vi "test-path-planner-basic.vi"() -> ()   [LabVIEW 2019]
uses:
  <vilib>/Rock Robotics/WPI/ThirdParty/MJansen/PathPlanner/TypeDef/PathPlannerTrajectoryState.ctl
  <vilib>/Rock Robotics/WPI/ThirdParty/JAS_Junk/TrajLib/TypeDef/TRANSLATION2D.ctl
  <vilib>/Rock Robotics/WPI/ThirdParty/JAS_Junk/TrajLib/TypeDef/ROTATION2D.ctl
  <vilib>/Rock Robotics/WPI/ThirdParty/MJansen/PathPlanner/TypeDef/PathPlannerPathConstraints.ctl
  <vilib>/Rock Robotics/WPI/ThirdParty/JAS_Junk/TrajLib/TypeDef/TRAJ_STATE.ctl
  <vilib>/Rock Robotics/WPI/ThirdParty/JAS_Junk/TrajLib/TypeDef/POSE2D.ctl
  <vilib>/Rock Robotics/WPI/ThirdParty/MJansen/PathPlanner/TypeDef/PathPlannerTrajectory.ctl
  <vilib>/Rock Robotics/WPI/ThirdParty/JAS_Junk/TrajLib/Util_ApproxEquals.vi
  <vilib>/Rock Robotics/WPI/ThirdParty/JAS_Junk/TrajLib/TrajectoryState_Equals.vi
  <vilib>/Rock Robotics/WPI/ThirdParty/JAS_Junk/TrajLib/Pose2d_Equals.vi
  <vilib>/Rock Robotics/WPI/ThirdParty/JAS_Junk/TrajLib/Translation2d_Equals.vi
  <vilib>/Rock Robotics/WPI/ThirdParty/JAS_Junk/TrajLib/Rotation2d_Equals.vi
  <vilib>/Rock Robotics/WPI/ThirdParty/JAS_Junk/TrajLib/Util_CalcDist.vi
  <vilib>/Rock Robotics/WPI/ThirdParty/MJansen/PathPlanner/PathPlanner24.lvlib
  <vilib>/Rock Robotics/WPI/ThirdParty/JAS_Junk/TrajLib/Trajectory_Library.lvlib
  <vilib>/Analysis/NI_AALBase.lvlib
panel:
  out "PathPlannerTrajectory":T1 {"States"."TargetHolonomicRotation"."SIN" format="%13.4f"; "States"."TargetHolonomicRotation"."COS" format="%13.4f"; "States"."TargetHolonomicRotation"."VALUE" format="%13.4f"; "States"."Heading"."SIN" format="%13.4f"; "States"."Heading"."COS" format="%13.4f"; "States"."Heading"."VALUE" format="%13.4f"; "States"."PositionMeters"."Y" format="%14.3f"; "States"."PositionMeters"."X" format="%14.3f"}
  in  "Tab Control":T6(tab)
  in  "jsonReadTrajFile":string="C:\\Shares\\github\\PathPlannerLabVIEW\\PathPlannerSandbox\\PathPlannerTestPath\\Javapath1.json"
  in  "stop":bool
  in  "Path FileName":string="C:\\Shares\\github\\PathPlannerLabVIEW\\PathPlannerSandbox\\PathPlannerTestPath\\jim1.PATH"
  out "LabVIEW path json read error":errorcluster
  in  "LabVIEW jsonWriteFile":string="C:\\Shares\\github\\PathPlannerLabVIEW\\PathPlannerSandbox\\PathPlannerTestPath\\LabVIEWpath1.json"
  out "Java File Read Error":errorcluster
  out "LabView Write\nJSON Error":errorcluster
  out "outPathPlannerStates":T2[](array[typedef]) {"TargetHolonomicRotation"."SIN" format="%13.4f"; "TargetHolonomicRotation"."COS" format="%13.4f"; "TargetHolonomicRotation"."VALUE" format="%13.4f"; "Heading"."SIN" format="%13.4f"; "Heading"."COS" format="%13.4f"; "Heading"."VALUE" format="%13.4f"; "PositionMeters"."Y" format="%14.3f"; "PositionMeters"."X" format="%14.3f"}
  in  "Down Button":bool
  in  "Up Button":bool
  in  "index":i32 step=20
  out "Java_TotalTime_Sec":dbl
  out "LabVIEW_TotalTime_Sec":dbl
  out "Jave and LabVIEW \nexactly equal":bool
  out "JavaStateCount":i32
  out "LabVIEWStateCount":i32
  out "States Check":bool[](array[boolean])
  out "JavaStates":T7[](array[typedef]) {"POSE"."ROTATION"."SIN" format="%13.4f"; "POSE"."ROTATION"."COS" format="%13.4f"; "POSE"."ROTATION"."VALUE" format="%13.4f"; "POSE"."TRANSLATION"."Y" format="%14.3f"; "POSE"."TRANSLATION"."X" format="%14.3f"}
  out "LabVIEWStates":T7[](array[typedef]) {"POSE"."ROTATION"."SIN" format="%13.4f"; "POSE"."ROTATION"."COS" format="%13.4f"; "POSE"."ROTATION"."VALUE" format="%13.4f"; "POSE"."TRANSLATION"."Y" format="%14.3f"; "POSE"."TRANSLATION"."X" format="%14.3f"}
  out "Differences":T7[](array[typedef]) {"POSE"."ROTATION"."SIN" format="%13.4f"; "POSE"."ROTATION"."COS" format="%13.4f"; "POSE"."ROTATION"."VALUE" format="%13.4f"; "POSE"."TRANSLATION"."Y" format="%14.3f"; "POSE"."TRANSLATION"."X" format="%14.3f"}
  out "max time diff":dbl
  out "max vel diff":dbl
  out "max accel diff":dbl
  out "max x diff":dbl
  out "max y diff":dbl
  out "max rot diff rad":dbl
  out "max curvature diff":dbl
  out "vel mean":dbl format="%0.6f"
  out "vel std dev":dbl format="%0.6f"
  out "accel mean":dbl format="%0.6f"
  out "accel std dev":dbl format="%0.6f"
  out "Java and LabVIEW \nwithin tolerance":bool
  in  "Tolerance":T7={"TimeSeconds"=0.15, "Velocity"=0.25, "Acceleration"=2.5, "POSE"={"TRANSLATION"={"X"=0.015, "Y"=0.015}, "ROTATION"={"VALUE"=0.01, "COS"=0.0, "SIN"=0.0}}, "Curvature"=1.4} {"POSE"."ROTATION"."SIN" format="%13.4f"; "POSE"."ROTATION"."COS" format="%13.4f"; "POSE"."ROTATION"."VALUE" format="%13.4f"; "POSE"."TRANSLATION"."Y" format="%14.3f"; "POSE"."TRANSLATION"."X" format="%14.3f"}
  out "XY SPLINE":cluster{dbl[], dbl[]}[](graph)
  out "XY Graph":cluster{dbl[], dbl[]}[](graph)
  out "Sample Graph":dbl[][](graph)
  out "LabVIEW Time Plot":cluster{dbl[], dbl[]}[](graph)
  out "Java Time Plot":cluster{dbl[], dbl[]}[](graph)
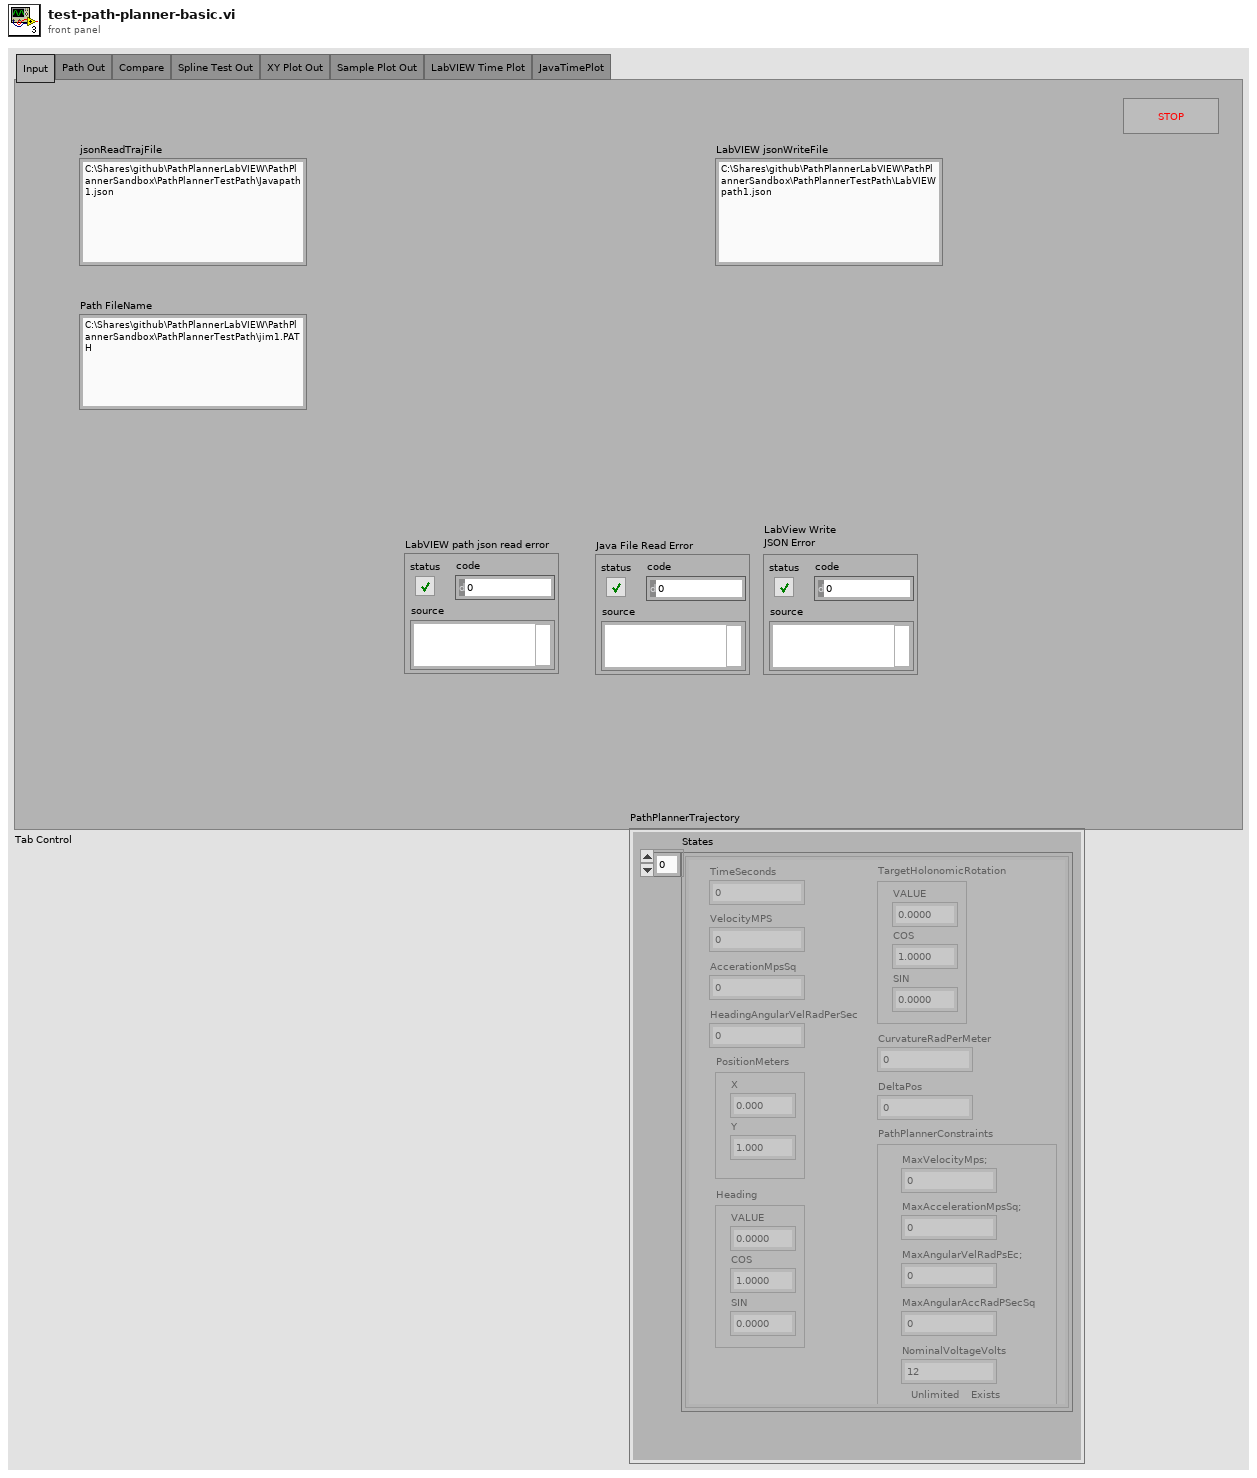
[diagram p1: front panel]
types:
  T1 = typedef "PathPlanner24.lvlib/PathPlannerTrajectory.ctl" = cluster{"States":T2[]}
  T2 = typedef "PathPlanner24.lvlib/PathPlannerTrajectoryState.ctl" = cluster{"TimeSeconds":dbl, "VelocityMPS":dbl, "AccerationMpsSq":dbl, "HeadingAngularVelRadPerSec":dbl, "PositionMeters":T3, "Heading":T4, "TargetHolonomicRotation":T4, "CurvatureRadPerMeter":dbl, "PathPlannerConstraints":T5, "DeltaPos":dbl}
  T3 = typedef "Trajectory_Library.lvlib/TRANSLATION2D.ctl" = cluster{"X":dbl, "Y":dbl}
  T4 = typedef "Trajectory_Library.lvlib/ROTATION2D.ctl" = cluster{"VALUE":dbl, "COS":dbl, "SIN":dbl}
  T5 = typedef "PathPlanner24.lvlib/PathPlannerPathConstraints.ctl" = cluster{"MaxVelocityMps;":dbl, "MaxAccelerationMpsSq;":dbl, "MaxAngularVelRadPsEc;":dbl, "MaxAngularAccRadPSecSq":dbl, "Exists":bool, "Unlimited":bool, "NominalVoltageVolts":dbl}
  T6 = enum32{"Input", "Path Out", "Compare", "Spline Test Out", "XY Plot Out", "Sample Plot Out", "LabVIEW Time Plot", "JavaTimePlot"}
  T7 = typedef "Trajectory_Library.lvlib/TRAJ_STATE.ctl" = cluster{"TimeSeconds":dbl, "Velocity":dbl, "Acceleration":dbl, "POSE":T8, "Curvature":dbl}
  T8 = typedef "Trajectory_Library.lvlib/POSE2D.ctl" = cluster{"TRANSLATION":T3, "ROTATION":T4}
  T9 = typedef "PathPlanner24.lvlib/PathPlannerPath.ctl" = cluster{"Reversed":bool, "RotationTargets":T10[], "ConstraintZones":T11[], "EventMarkers":T12[], "GlobalConstraints":T5, "GoalEndState":T15, "AllPoints":T16[], "Name":string, "Waypoints":T17[], "PointTowardsZones":T18[], "IdealStartingState":T19, "IsChoreoPath":bool, "PreventFlipping":bool}
  T10 = typedef "PathPlanner24.lvlib/PathPlannerRotationTarget.ctl" = cluster{"position":dbl, "rotation":T4, "Exists":bool}
  T11 = typedef "PathPlanner24.lvlib/PathPlannerConstraintsZone.ctl" = cluster{"minPosition":dbl, "maxPosition":dbl, "Constraints":T5, "Present":bool}
  T12 = typedef "PathPlanner24.lvlib/PathPlannerEventMarker.ctl" = cluster{"Position":dbl, "Command":T13, "TriggerName":string, "EndPosition":dbl}
  T13 = typedef "PathPlanner24.lvlib/PathPlannerCommandUtil.ctl" = cluster{"waitTime":dbl, "name":string, "pathName":string, "commands":cluster{"type":T14, "waitTime":dbl, "name":string, "pathName":string}[], "type":T14}
  T14 = typedef "PathPlanner24.lvlib/PathPlanner_CommandUtilType_ENUM.ctl" = enum16{"Unknown", "Wait", "Named", "Path", "Sequential", "Parallel", "Race", "Deadline"}
  T15 = typedef "PathPlanner24.lvlib/PathPlannerGoalEndState.ctl" = cluster{"VelocityMPS":dbl, "Rotation":T4}
  T16 = typedef "PathPlanner24.lvlib/PathPlannerPathPoint.ctl" = cluster{"Position":T3, "DistAlongPath":dbl, "MaxV":dbl, "Constraints":T5, "RotationTarget":T10, "WaypointRelativePos":dbl}
  T17 = typedef "PathPlanner24.lvlib/PathPlannerWaypoint.ctl" = cluster{"prevControl":T3, "anchor":T3, "nextControl":T3, "PrevExists":bool, "NextExists":bool}
  T18 = typedef "PathPlanner24.lvlib/PathPlannerPointTowardsZone.ctl" = cluster{"RotationOffset":T4, "Name":string, "TargetPosition":T3, "MinPosition":dbl, "MaxPosition":dbl}
  T19 = typedef "PathPlanner24.lvlib/PathPlannerIdealStartingState.ctl" = cluster{"VelocityMPS":dbl, "Rotation":T4}
  T20 = typedef "Trajectory_Library.lvlib/TRAJECTORY.ctl" = cluster{"TotalTImeSecs":dbl, "States":T7[]}
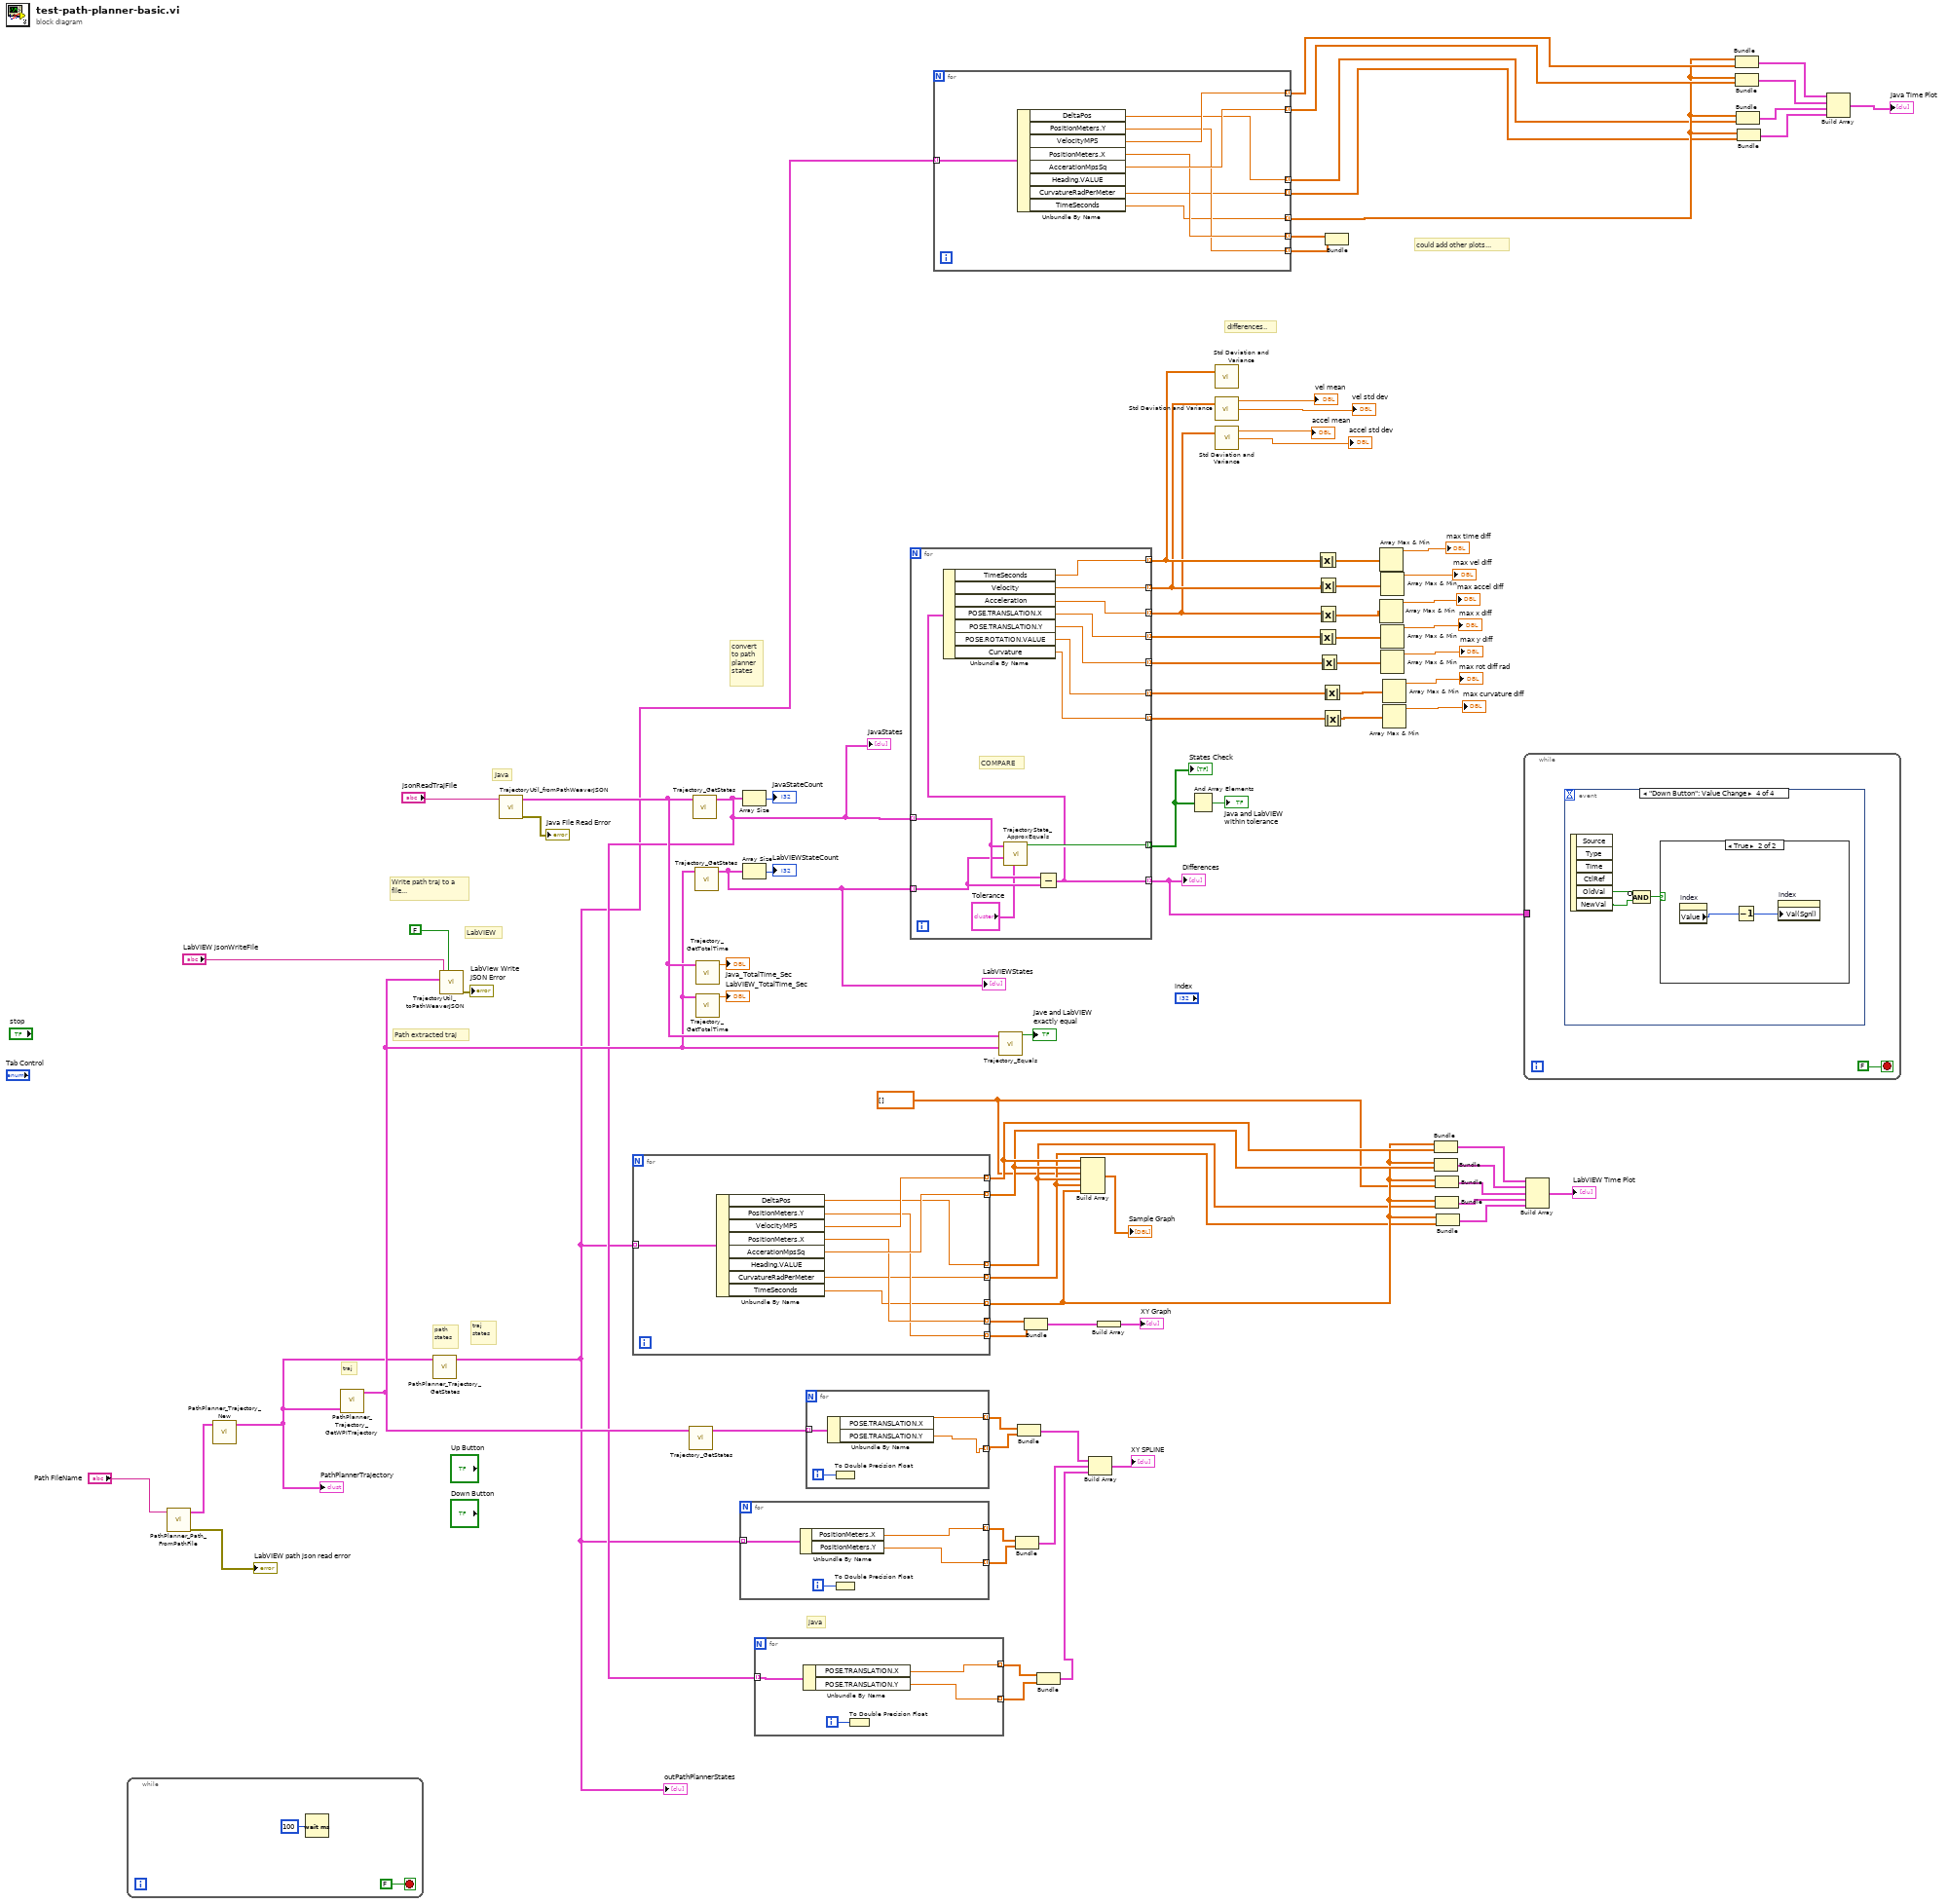
[diagram p0: block diagram]
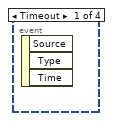
[diagram p2: hidden frame]
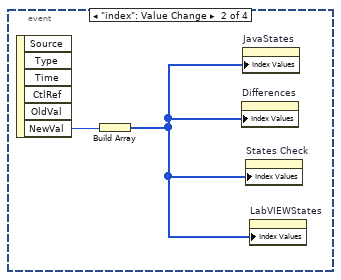
[diagram p3: hidden frame]
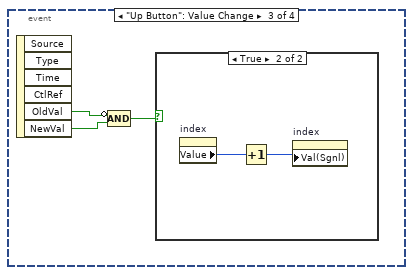
[diagram p4: hidden frame]
diagram:
  w2 = dbl[] [] ("element")
  # "Write path traj to a \nfile..."
  # "Path extracted traj"
  # "traj"
  # "traj\nstates"
  # "path\nstates"
  # "differences.."
  # "could add other plots..."
  # "convert\nto path\nplanner\nstates"
  # "java"
  # "LabVIEW"
  # "Java"
  n1 = while {
    stop <- FALSE stop-if-true
    n2 = Wait (ms)(milliseconds to wait=u32 100) -> ()  [unwired: 1 out]
  }
  n3 = call <vilib>:"PathPlanner_Path_FromPathFile.vi"("FileName"="Path FileName") -> ("error out"=→"LabVIEW path json read error":errorcluster, "PathPlannerPath"=w4:T9)  [unwired: 7 in, 2 out]
  n4 = call <vilib>:"PathPlanner_Trajectory_New.vi"("Path"=w4) -> ("PathPlannerTrajectory"=w3:T1)  [unwired: 9 in, 1 out]
  "PathPlannerTrajectory" <- w3
  n5 = call <vilib>:"PathPlanner_Trajectory_GetWPITrajectory.vi"("PathPlannerTrajectory"=w3) -> ("WPI TRAJECTORY"=w62:T20)  [unwired: 9 in, 1 out]
  n6 = call <vilib>:"PathPlanner_Trajectory_GetStates.vi"("PathPlannerTrajectory"=w3) -> ("PathPlannerStates"=w1:T2[])  [unwired: 10 in]
  "outPathPlannerStates" <- w1
  n7 = call <vilib>:"TrajectoryUtil_toPathWeaverJSON.vi"("AlwaysOverWrite"=FALSE, "inTRAJECTORY"=w62, "FileName"="LabVIEW jsonWriteFile") -> ("error out"=→"LabView Write\nJSON Error":errorcluster)  [unwired: 7 in, 1 out]
  n8 = call <vilib>:"TrajectoryUtil_fromPathWeaverJSON.vi"("FileName"="jsonReadTrajFile") -> ("error out"=→"Java File Read Error":errorcluster, "outTRAJECTORY"=w63:T20)  [unwired: 8 in, 1 out]
  n9 = for {
    tunnel: [w97] -> w31 mode=indexing
    tunnel: [w96] -> w30 mode=indexing
    tunnel: [w91] -> w28 mode=indexing
    tunnel: [w95] -> w86 mode=indexing
    tunnel: [w94] -> w85 mode=indexing
    tunnel: w1 -> [w93] mode=indexing
    tunnel: [w92] -> w27 mode=indexing
    tunnel: [w90] -> w29 mode=indexing
    n10 = Unbundle By Name(w93) -> ("DeltaPos"=w91:dbl, "PositionMeters.Y"=w94:dbl, "VelocityMPS"=w97:dbl, "PositionMeters.X"=w95:dbl, "AccerationMpsSq"=w96:dbl, "CurvatureRadPerMeter"=w92:dbl, "TimeSeconds"=w90:dbl)  [unwired: 1 out]
  }
  n11 = call <vilib>:"Trajectory_GetStates.vi"("TRAJECTORY"=w62) -> ("States"=w67:T7[])  [unwired: 10 in]
  n12 = call <vilib>:"Trajectory_GetStates.vi"("TRAJECTORY"=w63) -> ("States"=w10:T7[])  [unwired: 10 in]
  "JavaStates" <- w10
  n13 = call <vilib>:"Trajectory_GetStates.vi"("TRAJECTORY"=w62) -> ("States"=w59:T7[])  [unwired: 10 in]
  "LabVIEWStates" <- w59
  n14 = call <vilib>:"Trajectory_GetTotalTime.vi"("TRAJECTORY"=w63) -> ("TotalTime_Sec"=→"Java_TotalTime_Sec":dbl)  [unwired: 10 in]
  n15 = call <vilib>:"Trajectory_GetTotalTime.vi"("TRAJECTORY"=w62) -> ("TotalTime_Sec"=→"LabVIEW_TotalTime_Sec":dbl)  [unwired: 10 in]
  n16 = for {
    tunnel: [w100] -> w80 mode=indexing
    tunnel: w1 -> [w99] mode=indexing
    tunnel: [w98] -> w79 mode=indexing
    i -> [w101]
    n17 = Unbundle By Name(w99) -> ("PositionMeters.X"=w100:dbl, "PositionMeters.Y"=w98:dbl)
    n18 = To Double Precision Float(number=w101) -> ()  [unwired: 1 out]
  }
  n19 = Array Size(array=w10) -> (size(s)=→"JavaStateCount":i32)
  n20 = Array Size(array=w59) -> (size(s)=→"LabVIEWStateCount":i32)
  n21 = for {
    tunnel: [w104] -> w75 mode=indexing
    tunnel: w10 -> [w103] mode=indexing
    tunnel: [w102] -> w74 mode=indexing
    i -> [w105]
    n22 = Unbundle By Name(w103) -> ("POSE.TRANSLATION.X"=w104:dbl, "POSE.TRANSLATION.Y"=w102:dbl)
    n23 = To Double Precision Float(number=w105) -> ()  [unwired: 1 out]
  }
  n24 = for {
    tunnel: [w108] -> w82 mode=indexing
    tunnel: [w107] -> w81 mode=indexing
    tunnel: w67 -> [w106] mode=indexing
    i -> [w109]
    n25 = Unbundle By Name(w106) -> ("POSE.TRANSLATION.X"=w108:dbl, "POSE.TRANSLATION.Y"=w107:dbl)
    n26 = To Double Precision Float(number=w109) -> ()  [unwired: 1 out]
  }
  n27 = for {
    tunnel: w10 -> [w120] mode=indexing
    tunnel: w59 -> [w119] mode=indexing
    tunnel: [w121] -> w9 mode=indexing
    tunnel: [w118] -> w58 mode=indexing
    tunnel: [w117] -> w39 mode=indexing
    tunnel: [w116] -> w38 mode=indexing
    tunnel: [w115] -> w37 mode=indexing
    tunnel: [w114] -> w54 mode=indexing
    tunnel: [w113] -> w55 mode=indexing
    tunnel: [w112] -> w56 mode=indexing
    tunnel: [w111] -> w57 mode=indexing
    # "COMPARE"
    n28 = call "TrajectoryState_ApproxEquals.vi"("Tolerance"="Tolerance", "Other TRAJ_STATE"=w119, "TRAJ_STATE"=w120) -> ("Equals"=w121:bool)  [unwired: 8 in]
    n29 = Subtract(x=w120, y=w119) -> (x-y=w118:T7)
    n30 = Unbundle By Name(w118) -> ("TimeSeconds"=w117:dbl, "Velocity"=w116:dbl, "Acceleration"=w115:dbl, "POSE.TRANSLATION.X"=w114:dbl, "POSE.TRANSLATION.Y"=w113:dbl, "POSE.ROTATION.VALUE"=w112:dbl, "Curvature"=w111:dbl)
  }
  "States Check" <- w9
  "Differences" <- w58
  n31 = for {
    tunnel: [w129] -> w19 mode=indexing
    tunnel: [w128] -> w18 mode=indexing
    tunnel: [w123] -> w16 mode=indexing
    tunnel: [w127] -> w21 mode=indexing
    tunnel: [w126] -> w20 mode=indexing
    tunnel: w1 -> [w125] mode=indexing
    tunnel: [w124] -> w15 mode=indexing
    tunnel: [w122] -> w17 mode=indexing
    n32 = Unbundle By Name(w125) -> ("DeltaPos"=w123:dbl, "PositionMeters.Y"=w126:dbl, "VelocityMPS"=w129:dbl, "PositionMeters.X"=w127:dbl, "AccerationMpsSq"=w128:dbl, "CurvatureRadPerMeter"=w124:dbl, "TimeSeconds"=w122:dbl)  [unwired: 1 out]
  }
  n33 = call <vilib>:"Trajectory_Equals.vi"("other TRAJECTORY"=w62, "TRAJECTORY"=w63) -> ("Equals"=→"Jave and LabVIEW \nexactly equal":bool)  [unwired: 9 in]
  n34 = Bundle(w80, w79) -> (w77:cluster{dbl[], dbl[]})  [unwired: 1 in]
  n35 = Bundle(w82, w81) -> (w78:cluster{dbl[], dbl[]})  [unwired: 1 in]
  n36 = Bundle(w86, w85) -> (w84:cluster{dbl[], dbl[]})  [unwired: 1 in]
  n37 = Bundle(w75, w74) -> (w73:cluster{dbl[], dbl[]})  [unwired: 1 in]
  n38 = Build Array(w31, w30, w2, w28, w27, w29) -> (→"Sample Graph":dbl[][])
  n39 = Build Array(w78, w77, w73) -> (→"XY SPLINE":cluster{dbl[], dbl[]}[])
  n40 = Build Array(w84) -> (→"XY Graph":cluster{dbl[], dbl[]}[])
  n41 = And Array Elements(Boolean array=w9) -> (logical AND=→"Java and LabVIEW \nwithin tolerance":bool)
  n42 = call <vilib>:"Std Deviation and Variance.vi"("X"=w39) -> ()  [unwired: 1 in, 3 out]
  n43 = call <vilib>:"Std Deviation and Variance.vi"("X"=w38) -> ("mean"=→"vel mean":dbl, "standard deviation"=→"vel std dev":dbl)  [unwired: 1 in, 1 out]
  n44 = call <vilib>:"Std Deviation and Variance.vi"("X"=w37) -> ("mean"=→"accel mean":dbl, "standard deviation"=→"accel std dev":dbl)  [unwired: 1 in, 1 out]
  n45 = Absolute Value(x=w39) -> (abs(x)=w47:dbl[])
  n46 = Absolute Value(x=w54) -> (abs(x)=w50:dbl[])
  n47 = Absolute Value(x=w38) -> (abs(x)=w48:dbl[])
  n48 = Absolute Value(x=w37) -> (abs(x)=w49:dbl[])
  n49 = Absolute Value(x=w55) -> (abs(x)=w51:dbl[])
  n50 = Absolute Value(x=w56) -> (abs(x)=w52:dbl[])
  n51 = Absolute Value(x=w57) -> (abs(x)=w53:dbl[])
  n52 = Bundle(w21, w20) -> ()  [unwired: 1 in, 1 out]
  n53 = Array Max & Min(array=w47) -> (max value=→"max time diff":dbl)  [unwired: 3 out]
  n54 = Array Max & Min(array=w49) -> (max value=→"max accel diff":dbl)  [unwired: 3 out]
  n55 = Array Max & Min(array=w48) -> (max value=→"max vel diff":dbl)  [unwired: 3 out]
  n56 = Array Max & Min(array=w50) -> (max value=→"max x diff":dbl)  [unwired: 3 out]
  n57 = Array Max & Min(array=w51) -> (max value=→"max y diff":dbl)  [unwired: 3 out]
  n58 = Array Max & Min(array=w52) -> (max value=→"max rot diff rad":dbl)  [unwired: 3 out]
  n59 = Array Max & Min(array=w53) -> (max value=→"max curvature diff":dbl)  [unwired: 3 out]
  n60 = Bundle(w29, w31) -> (w26:cluster{dbl[], dbl[]})  [unwired: 1 in]
  n61 = Bundle(w29, w30) -> (w25:cluster{dbl[], dbl[]})  [unwired: 1 in]
  n62 = Bundle(w29, "element"=w2) -> (w24:cluster{dbl[], "element":dbl[]})  [unwired: 1 in]
  n63 = Bundle(w29, w28) -> (w23:cluster{dbl[], dbl[]})  [unwired: 1 in]
  n64 = Bundle(w29, w27) -> (w22:cluster{dbl[], dbl[]})  [unwired: 1 in]
  n65 = while {
    tunnel: w58 -> [_]
    stop <- FALSE stop-if-true
    n66 = event shown="[3] \"Down Button\": Value Change" {
      selector: _ -> [_ _ _ _]
      dyn-events: _ -> [_ _ _ _]
      timeout: _ -> [_ _ _ _]
      event Timeout {
        n67 = event-data() -> ()  [unwired: 1 in, 3 out]
      }
      event "index": Value Change {
        n68 = event-data() -> ("NewVal"=w132:i32)  [unwired: 1 in, 5 out]
        n69 = Build Array(w132) -> (w131:i32[])
        n70 = property on="Differences" class="Arr (strict)"("Index Values"=w131) -> ()  [unwired: 2 in, 2 out]
        n71 = property on="JavaStates" class="Arr (strict)"("Index Values"=w131) -> ()  [unwired: 2 in, 2 out]
        n72 = property on="States Check" class="Arr (strict)"("Index Values"=w131) -> ()  [unwired: 2 in, 2 out]
        n73 = property on="LabVIEWStates" class="Arr (strict)"("Index Values"=w131) -> ()  [unwired: 2 in, 2 out]
      }
      event "Up Button": Value Change {
        n74 = event-data() -> ("OldVal"=w135:bool, "NewVal"=w134:bool)  [unwired: 1 in, 4 out]
        n75 = Compound Arithmetic op=AND(invert w135, w134) -> (w133:bool)
        n76 = case shown="True" w133 {
          frame False {
          }
          frame True {
            n77 = property on="index" class="DigNum (strict)"() -> ("Value"=w136:i32)  [unwired: 2 in, 2 out]
            n78 = Increment(x=w136) -> (x+1=w137:i32)
            n79 = property on="index" class="DigNum (strict)"("Val(Sgnl)"=w137) -> ()  [unwired: 2 in, 2 out]
          }
        }
      }
      event "Down Button": Value Change {
        n80 = event-data() -> ("OldVal"=w139:bool, "NewVal"=w138:bool)  [unwired: 1 in, 4 out]
        n81 = Compound Arithmetic op=AND(invert w139, w138) -> (w140:bool)
        n82 = case shown="True" w140 {
          frame False {
          }
          frame True {
            n83 = property on="index" class="DigNum (strict)"() -> ("Value"=w141:i32)  [unwired: 2 in, 2 out]
            n84 = Decrement(x=w141) -> (x-1=w142:i32)
            n85 = property on="index" class="DigNum (strict)"("Val(Sgnl)"=w142) -> ()  [unwired: 2 in, 2 out]
          }
        }
      }
    }
  }
  n86 = Build Array(w26, w25, w24, w23, w22) -> (→"LabVIEW Time Plot":cluster{dbl[], "element":dbl[]}[])
  n87 = Bundle(w17, w19) -> (w14:cluster{dbl[], dbl[]})  [unwired: 1 in]
  n88 = Bundle(w17, w18) -> (w13:cluster{dbl[], dbl[]})  [unwired: 1 in]
  n89 = Bundle(w17, w16) -> (w12:cluster{dbl[], dbl[]})  [unwired: 1 in]
  n90 = Bundle(w17, w15) -> (w11:cluster{dbl[], dbl[]})  [unwired: 1 in]
  n91 = Build Array(w14, w13, w12, w11) -> (→"Java Time Plot":cluster{dbl[], dbl[]}[])
